vi "Get Board HW Entry by id.vi"(10 "board":u32, 11 "hw_data in":T3) -> (1 "board resource out":T1, 2 "key not found?":bool, 3 "hw_data out":T3)   [LabVIEW 2020, in "AIM664LV.lvlib"]
uses:
  AIM664LV.lvlib
  _controls/hwEntry_data.ctl
  _controls/hwEntryBoardHandleMap.ctl
  _controls/hwEntryBoardResource.ctl
  _controls/hwEntryPortResource.ctl
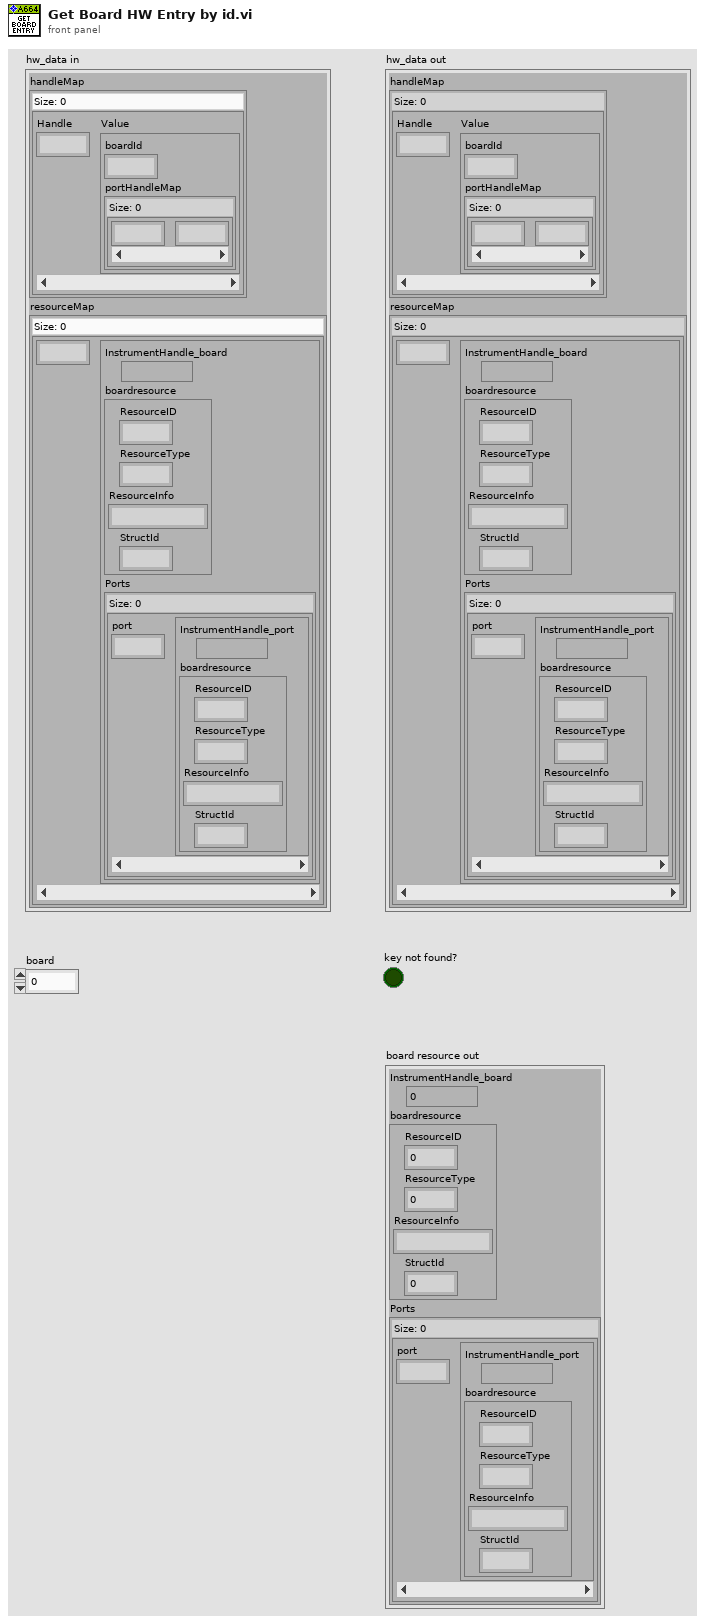
[diagram p1: front panel]
types:
  T1 = typedef "AIM664LV.lvlib/hwEntryBoardResource.ctl" = cluster{"InstrumentHandle_board":u32, "boardresource":cluster{"ResourceID":u32, "ResourceType":u32, "ResourceInfo":string, "StructId":u32}, "Ports":map{u32, T2}}
  T2 = typedef "AIM664LV.lvlib/hwEntryPortResource.ctl" = cluster{"InstrumentHandle_port":u32, "boardresource":cluster{"ResourceID":u32, "ResourceType":u32, "ResourceInfo":string, "StructId":u32}}
  T3 = typedef "AIM664LV.lvlib/hwEntry_data.ctl" = cluster{"handleMap":map{u32, T4}, "resourceMap":map{u32, T1}}
  T4 = typedef "AIM664LV.lvlib/hwEntryBoardHandleMap.ctl" = cluster{"boardId":u32, "portHandleMap":map{u32, u32}}
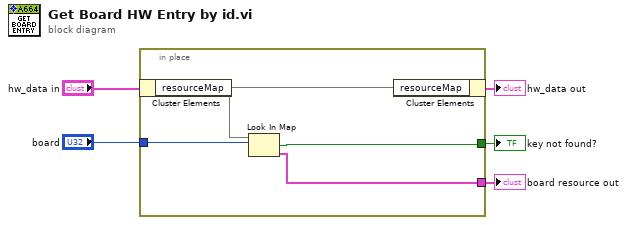
[diagram p0: block diagram]
diagram:
  n1 = in-place {
    in-place-border: "board" -> [w8]
    in-place-border: [w7] -> w1
    in-place-border: [w6] -> w2
    n2 = in-place-cluster #1("hw_data in") -> ("resourceMap"=w9:map{u32, T1})
    n3 = Look In Map(map=w9, key=w8) -> (key not found?=w6:bool, value=w7:T1)  [unwired: 1 in]
    n4 = in-place-cluster #1("resourceMap"=w9) -> (→"hw_data out":T3)
  }
  "key not found?" <- w2
  "board resource out" <- w1
